vi "Untitled 2.vi"(8 "error in (no error)":errorcluster) -> ()   [LabVIEW 2015]
uses:
  Camera Types.ctl
  <vilib>/Rock Robotics/WPI/Camera/WPI_CameraImageSize.ctl
  <vilib>/Rock Robotics/WPI/Camera/WPI_CameraWhite Balance Values.ctl
  <vilib>/Rock Robotics/WPI/Camera/WPI_CameraExposure Values.ctl
  <vilib>/Rock Robotics/WPI/Camera/WPI_CameraFrameRate.ctl
  Global 2.vi
  Robot Global Data.vi
  Global 1.vi
  <vilib>/vision/NI_Vision_Development_Module.lvlib
panel:
  in  "Cluster":T1={"Hue"={105.0, 150.0}, "Sat"={191.0, 255.0}, "Val"={173.0, 255.0}}
  in  "Image Size":T2=enum."320x240"
  out "Original Image":T3(plugin-control)
  out "Masked":T3(plugin-control)
  out "Qualified Particles":i32
  out "Sorted Particle Scores":T4(array[cluster]) {"Moment Factor" format="%#_3g"; "Aspect Ratio" format="%#_3g"; "Area to CH" format="%#_3g"; "X" format="%#_3g"; "Y" format="%#_3g"}
  in  "Annotate":bool=TRUE
  in  "Annotation Limit":dbl=75.0
  out "Detected Targets":T5(array[cluster]) {"Normalized Rect"."Numeric 5" format="%#_2g"; "Normalized Rect"."Numeric 3" format="%#_2g"; "Normalized Rect"."Numeric 2" format="%#_2g"; "Normalized Rect"."Numeric" format="%#_2g"}
  in  "Aspect Ratio Fudge Factor":dbl=1.0
  out "Highest Avg Score":dbl format="%#_3g"
  in  "Min Score Threshold":i32=70
  in  "Camera Type":T6=enum."MS HD3000 square"
  in  "Emphasize Limit Tests":bool=TRUE
  in  "Std Devs for Calibration":cluster{"H":dbl, "S":dbl, "V":dbl}={"H"=4.0, "S"=6.0, "V"=6.0}
  # "Density Profile"
  # "x"
  # "y"
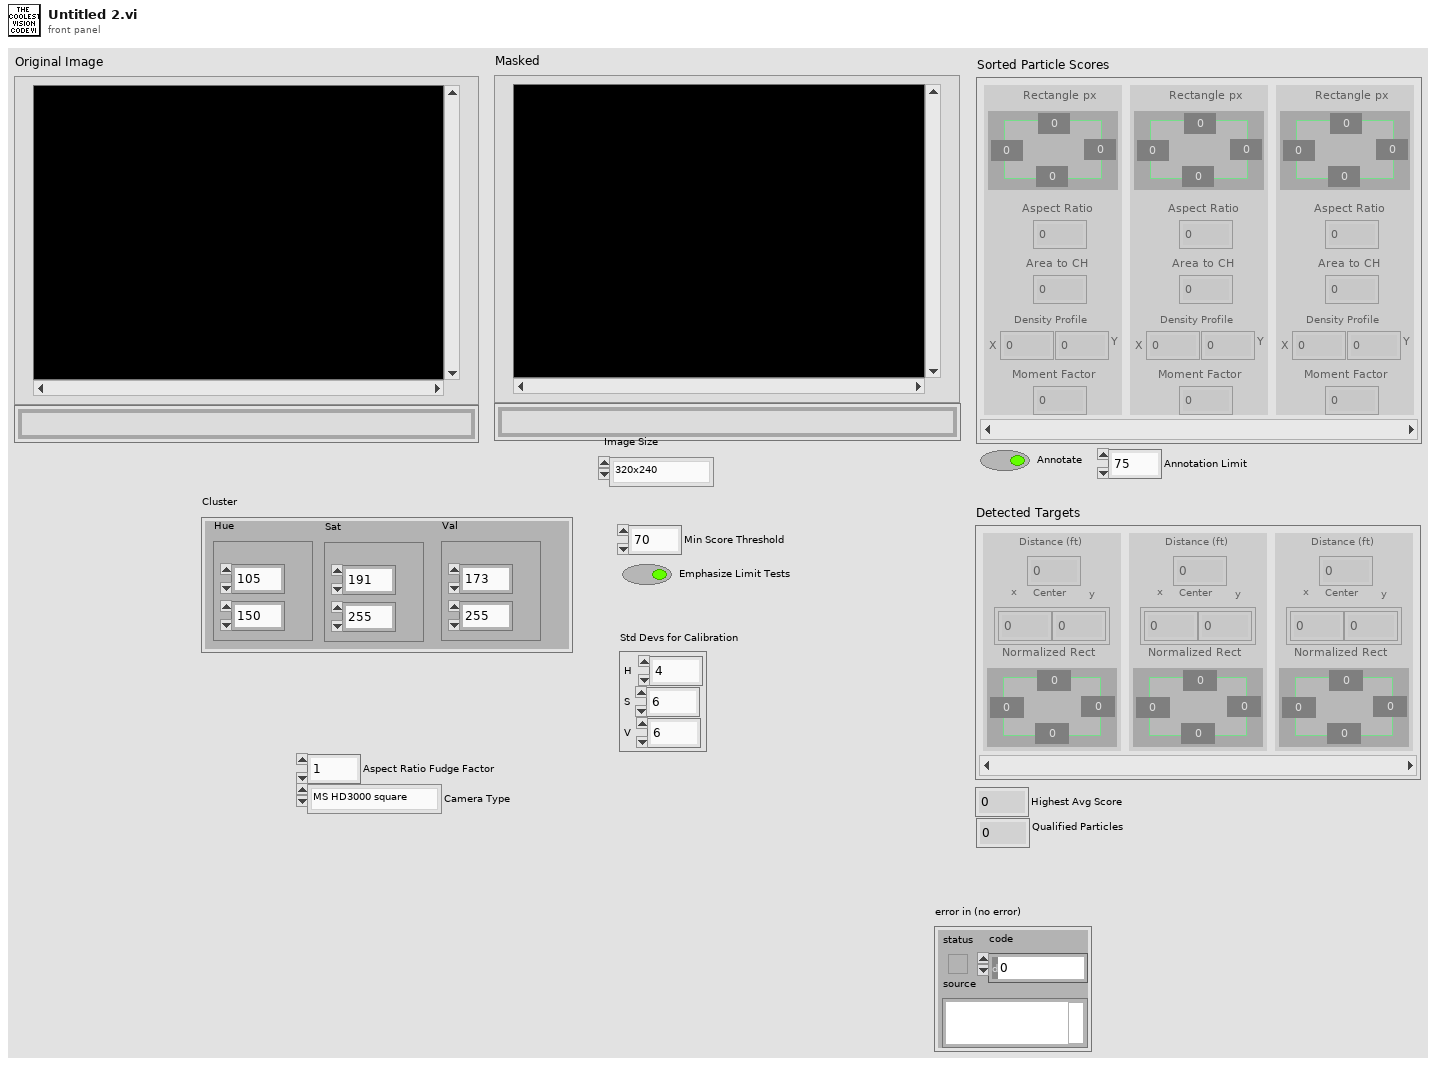
[diagram p1: front panel]
types:
  T1 = cluster{"Hue":cluster{dbl, dbl}, "Sat":cluster{dbl, dbl}, "Val":cluster{dbl, dbl}}
  T2 = typedef "WPI_CameraImageSize.ctl" = enum16{"640x480", "320x240", "160x120", "Custom"}
  T3 = typedef "IMAQ Image.ctl" = refnum<image>
  T4 = cluster{"Rectangle px":cluster{"Numeric":dbl, "Numeric 2":dbl, "Numeric 3":dbl, "Numeric 5":dbl}, "Aspect Ratio":dbl, "Area to CH":dbl, "X":dbl, "Y":dbl, "Moment Factor":dbl}[]
  T5 = cluster{"Distance (ft)":dbl, "Center":cluster{dbl, dbl}, "Normalized Rect":cluster{"Numeric":dbl, "Numeric 2":dbl, "Numeric 3":dbl, "Numeric 5":dbl}}[]
  T6 = typedef "Camera Types.ctl" = enum16{"206", "1011", "1013", "MS HD3000 square", "MS HD3000 640x480"}
  T7 = typedef "WPI_CameraFrameRate.ctl" = u32
  T8 = typedef "WPI_CameraExposure Values.ctl" = enum16{"Auto", "Flicker-free 50 Hz", "Flicker-free 60 Hz", "Hold current", "Custom"}
  T9 = typedef "WPI_CameraWhite Balance Values.ctl" = enum16{"Auto", "Fixed indoor", "Fixed outdoor 1", "Fixed outdoor 2", "Fixed fluorescent 1", "Fixed fluorescent 2", "Hold current", "Custom"}
  T10 = typedef "Particle Parameters" = i32
  T11 = typedef "Image Type" = u32
  T12 = typedef "WPI_CameraDevRef.ctl" = cluster{"Camera Address":string, "CameraStatus":errorcluster}
  T13 = cluster{cluster{dbl, dbl}, cluster{dbl, dbl}, cluster{dbl, dbl}}
  T14 = cluster{"Bounding box":cluster{"left":dbl, "top":dbl, "right":dbl, "bottom":dbl}, "Aspect Ratio":dbl, "Area to CH":dbl, "X Mask":dbl, "Y Mask":dbl, "Moment":dbl}[]
  T15 = cluster{"Rectangle":cluster{"Numeric":dbl, "Numeric 2":dbl, "Numeric 3":dbl, "Numeric 5":dbl}, "L":dbl, "Area to CH":dbl, "X":dbl, "Y":dbl, "Moment Factor":dbl}[]
  T16 = cluster{"Found Targets[0]":cluster{"Distance (ft)":dbl, "Center":cluster{dbl, dbl}, "Normalized Rect":cluster{"Numeric":dbl, "Numeric 2":dbl, "Numeric 3":dbl, "Numeric 5":dbl}}, "Found Targets[1]":cluster{"Distance (ft)":dbl, "Center":cluster{dbl, dbl}, "Normalized Rect":cluster{"Numeric":dbl, "Numeric 2":dbl, "Numeric 3":dbl, "Numeric 5":dbl}}, "Found Targets[2]":cluster{"Distance (ft)":dbl, "Center":cluster{dbl, dbl}, "Normalized Rect":cluster{"Numeric":dbl, "Numeric 2":dbl, "Numeric 3":dbl, "Numeric 5":dbl}}, "Found Targets[3]":cluster{"Distance (ft)":dbl, "Center":cluster{dbl, dbl}, "Normalized Rect":cluster{"Numeric":dbl, "Numeric 2":dbl, "Numeric 3":dbl, "Numeric 5":dbl}}, "Found Targets[4]":cluster{"Distance (ft)":dbl, "Center":cluster{dbl, dbl}, "Normalized Rect":cluster{"Numeric":dbl, "Numeric 2":dbl, "Numeric 3":dbl, "Numeric 5":dbl}}, "Found Targets[5]":cluster{"Distance (ft)":dbl, "Center":cluster{dbl, dbl}, "Normalized Rect":cluster{"Numeric":dbl, "Numeric 2":dbl, "Numeric 3":dbl, "Numeric 5":dbl}}, "Found Targets[6]":cluster{"Distance (ft)":dbl, "Center":cluster{dbl, dbl}, "Normalized Rect":cluster{"Numeric":dbl, "Numeric 2":dbl, "Numeric 3":dbl, "Numeric 5":dbl}}, "Found Targets[7]":cluster{"Distance (ft)":dbl, "Center":cluster{dbl, dbl}, "Normalized Rect":cluster{"Numeric":dbl, "Numeric 2":dbl, "Numeric 3":dbl, "Numeric 5":dbl}}, "Found Targets[8]":cluster{"Distance (ft)":dbl, "Center":cluster{dbl, dbl}, "Normalized Rect":cluster{"Numeric":dbl, "Numeric 2":dbl, "Numeric 3":dbl, "Numeric 5":dbl}}}
  T17 = cluster{"Distance (ft)":dbl, "Center":cluster{dbl, dbl}, "Normalized Rect":cluster{"Numeric":dbl, "Numeric 2":dbl, "Numeric 3":dbl, "Numeric 5":dbl}}
  T18 = cluster{"Numeric":dbl, "Numeric 2":dbl, "Numeric 3":dbl, "Numeric 5":dbl}
  T19 = cluster{"Distance (ft)":dbl, cluster{dbl, dbl}, "Normalized Rect":cluster{"Numeric":dbl, "Numeric 2":dbl, "Numeric 3":dbl, "Numeric 5":dbl}}
  T20 = cluster{cluster{"Distance (ft)":dbl, cluster{dbl, dbl}, "Normalized Rect":cluster{"Numeric":dbl, "Numeric 2":dbl, "Numeric 3":dbl, "Numeric 5":dbl}}, cluster{"Distance (ft)":dbl, cluster{dbl, dbl}, "Normalized Rect":cluster{"Numeric":dbl, "Numeric 2":dbl, "Numeric 3":dbl, "Numeric 5":dbl}}, cluster{"Distance (ft)":dbl, cluster{dbl, dbl}, "Normalized Rect":cluster{"Numeric":dbl, "Numeric 2":dbl, "Numeric 3":dbl, "Numeric 5":dbl}}, "Found Targets[3]":cluster{"Distance (ft)":dbl, "Center":cluster{dbl, dbl}, "Normalized Rect":cluster{"Numeric":dbl, "Numeric 2":dbl, "Numeric 3":dbl, "Numeric 5":dbl}}, "Found Targets[4]":cluster{"Distance (ft)":dbl, "Center":cluster{dbl, dbl}, "Normalized Rect":cluster{"Numeric":dbl, "Numeric 2":dbl, "Numeric 3":dbl, "Numeric 5":dbl}}, "Found Targets[5]":cluster{"Distance (ft)":dbl, "Center":cluster{dbl, dbl}, "Normalized Rect":cluster{"Numeric":dbl, "Numeric 2":dbl, "Numeric 3":dbl, "Numeric 5":dbl}}, "Found Targets[6]":cluster{"Distance (ft)":dbl, "Center":cluster{dbl, dbl}, "Normalized Rect":cluster{"Numeric":dbl, "Numeric 2":dbl, "Numeric 3":dbl, "Numeric 5":dbl}}, "Found Targets[7]":cluster{"Distance (ft)":dbl, "Center":cluster{dbl, dbl}, "Normalized Rect":cluster{"Numeric":dbl, "Numeric 2":dbl, "Numeric 3":dbl, "Numeric 5":dbl}}, "Found Targets[8]":cluster{"Distance (ft)":dbl, "Center":cluster{dbl, dbl}, "Normalized Rect":cluster{"Numeric":dbl, "Numeric 2":dbl, "Numeric 3":dbl, "Numeric 5":dbl}}}
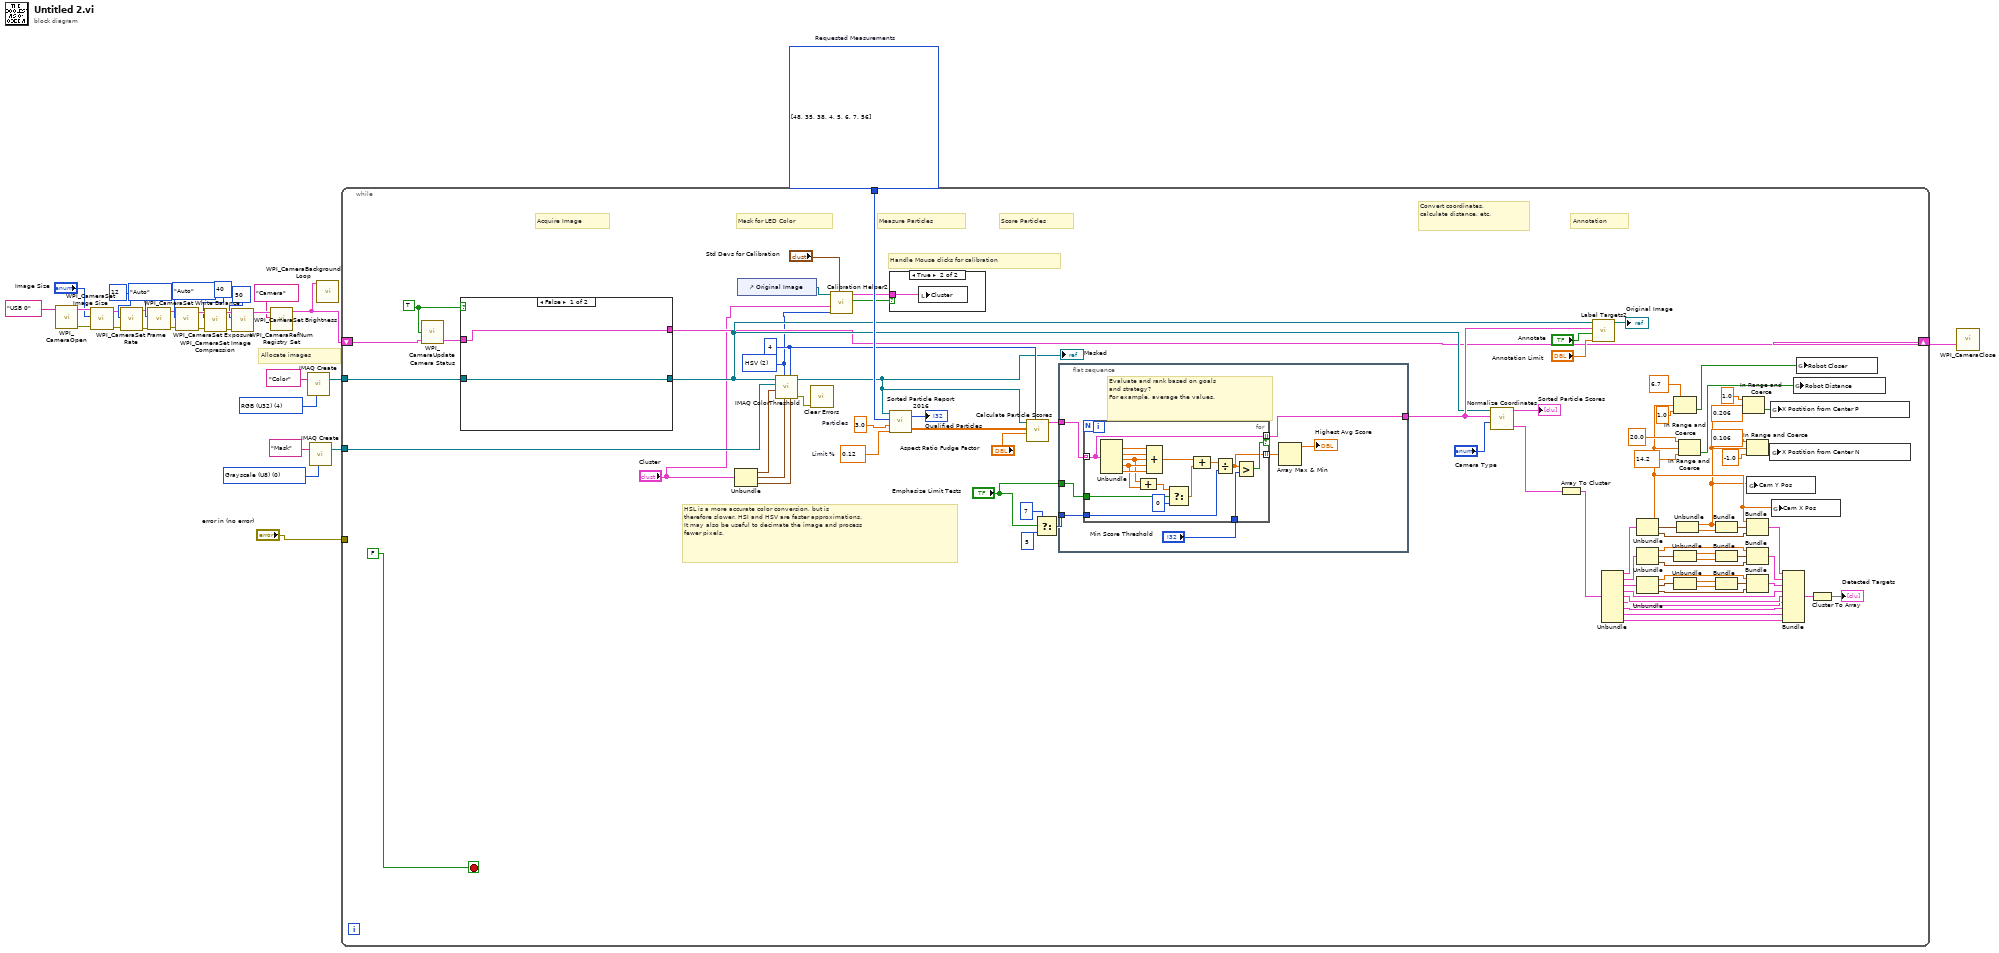
[diagram p0: block diagram]
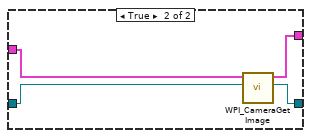
[diagram p3: hidden frame]
diagram:
  w25 = T10[] [48, 35, 38, 4, 5, 6, 7, 56] items=["Center of Mass X", "Center of Mass Y", "First Pixel X", "First Pixel Y", "Bounding Rect Left", "Bounding Rect Top", "Bounding Rect Right", "Bounding Rect Bottom", "Max Feret Diameter Start X", "Max Feret Diameter Start Y", "Max Feret Diameter End X", "Max Feret Diameter End Y", "Max Horiz. Segment Length Left", "Max Horiz. Segment Length Right", "Max Horiz. Segment Length Row", "-", "Bounding Rect Width", "Bounding Rect Height", "Bounding Rect Diagonal", "Perimeter", "Convex Hull Perimeter", "Holes' Perimeter", "Max Feret Diameter", "Equivalent Ellipse Major Axis", "Equivalent Ellipse Minor Axis", "Equivalent Ellipse Minor Axis (Feret)", "Equivalent Rect Long Side", "Equivalent Rect Short Side", "Equivalent Rect Diagonal", "Equivalent Rect Short Side (Feret)", "Average Horiz. Segment Length", "Average Vert. Segment Length", "Hydraulic Radius", "Waddel Disk Diameter", "-", "Area", "Holes' Area", "Particle & Holes' Area", "Convex Hull Area", "Image Area", "-", "Number of Holes", "Number of Horiz. Segments", "Number of Vert. Segments", "-", "Orientation", "Max Feret Diameter Orientation", "-", "% Area/Image Area", "% Area/(Particle & Holes' Area)", "Ratio of Equivalent Ellipse Axes", "Ratio of Equivalent Rect Sides", "-", "Elongation Factor", "Compactness Factor", "Heywood Circularity Factor", "Type Factor", "-", "Sum X", "Sum Y", "Sum XX", "Sum XY", "Sum YY", "Sum XXX", "Sum XXY", "Sum XYY", "Sum YYY", "-", "Moment of Inertia XX", "Moment of Inertia XY", "Moment of Inertia YY", "Moment of Inertia XXX", "Moment of Inertia XXY", "Moment of Inertia XYY", "Moment of Inertia YYY", "Norm. Moment of Inertia XX", "Norm. Moment of Inertia XY", "Norm. Moment of Inertia YY", "Norm. Moment of Inertia XXX", "Norm. Moment of Inertia XXY", "Norm. Moment of Inertia XYY", "Norm. Moment of Inertia YYY", "Hu Moment 1", "Hu Moment 2", "Hu Moment 3", "Hu Moment 4", "Hu Moment 5", "Hu Moment 6", "Hu Moment 7"]  # Requested Measurements
  w28 = T11 0 items=["Grayscale (U8)", "Grayscale (I16)", "Grayscale (SGL)", "Complex (CSG)", "RGB (U32)", "HSL (U32)", "RGB (U64)", "Grayscale (U16)"] ("Image Type")
  w30 = T11 4 items=["Grayscale (U8)", "Grayscale (I16)", "Grayscale (SGL)", "Complex (CSG)", "RGB (U32)", "HSL (U32)", "RGB (U64)", "Grayscale (U16)"] ("Image Type")
  # "Allocate images"
  n1 = call <vilib>:"WPI_CameraOpen.vi"("Camera Address"="USB 0") -> ("error out"=w11:errorcluster, "CameraDevRef"=w24:T12)  [unwired: 9 in]
  n2 = call <vilib>:"WPI_CameraSet Image Size.vi"("error in (no error)"=w11, "Image Size"="Image Size", "CameraDevRef"=w24) -> ("error out"=w10:errorcluster, "CameraDevRef Out"=w19:T12)  [unwired: 1 in, 6 out]
  n3 = call <vilib>:"WPI_CameraSet Frame Rate.vi"("error in (no error)"=w10, "Frame Rate (fps)"=T7 12, "CameraDevRef"=w19) -> ("error out"=w9:errorcluster, "CameraDevRef Out"=w17:T12)  [unwired: 7 out]
  n4 = call <vilib>:"WPI_CameraSet White Balance.vi"("error in (no error)"=w9, "White Balance"=WPI_CameraWhite_Balance_Values."Auto", "CameraDevRef"=w17) -> ("error out"=w8:errorcluster, "CameraDevRef Out"=w18:T12)  [unwired: 1 in, 6 out]
  n5 = call <vilib>:"WPI_CameraSet Exposure.vi"("error in (no error)"=w8, "Exposure"=WPI_CameraExposure_Values."Auto", "CameraDevRef"=w18) -> ("error out"=w7:errorcluster, "CameraDevRef Out"=w15:T12)  [unwired: 1 in, 6 out]
  n6 = call <vilib>:"WPI_CameraSet Image Compression.vi"("error in (no error)"=w7, "Compression"=40, "CameraDevRef"=w15) -> ("error out"=w6:errorcluster, "CameraDevRef Out"=w16:T12)  [unwired: 7 out]
  n7 = call <vilib>:"WPI_CameraSet Brightness.vi"("error in (no error)"=w6, "Brightness"=50, "CameraDevRef"=w16) -> ("CameraDevRef Out"=w4:T12)  [unwired: 8 out]
  n8 = call <vilib>:"WPI_CameraRefNum Registry Set.vi"("refnum name"="Camera", "CameraDevRef"=w4) -> ("CameraDevRef"=w1:T12)  [unwired: 8 in, 1 out]
  n9 = call "IMAQ Create"("Image Name"="Color", "Image Type"=w30) -> ("New Image"=w29:T3)  [unwired: 2 in, 2 out]
  n10 = call "IMAQ Create"("Image Name"="Mask", "Image Type"=w28) -> ("New Image"=w26:T3)  [unwired: 2 in, 2 out]
  n11 = call <vilib>:"WPI_CameraBackground Loop.vi"("CameraDevRef"=w1) -> ()  [unwired: 11 in]
  n12 = while {
    tunnel: w29 -> [w114]
    tunnel: w26 -> [w112]
    tunnel: w25 -> [w108]
    tunnel: "error in (no error)" -> [_]
    shift-right: [w85] -> w2
    shift-left: w1 -> [w84]
    stop <- FALSE stop-if-true
    w86 = TRUE
    w101 = 4 ("Replace Value")
    w104 = 0.12  # Limit %
    w107 = 3.0  # Particles
    w79 = u16 2 items=["RGB", "HSL", "HSV", "HSI"] ("Color Mode")
    # "Handle Mouse clicks for calibration"
    # "Measure Particles"
    # "Convert coordinates,\ncalculate distance, etc."
    # "Annotation"
    # "Score Particles"
    # "Mask for LED Color"
    # "Acquire Image"
    # "HSL is a more accurate color conversion, but is\ntherefore slower. HSI and HSV are faster approximations.\nIt may also be useful to decimate the image and process\nfewer pixels."
    n13 = call <vilib>:"WPI_CameraUpdate Camera Status.vi"("CameraDevRef In"=w84, "Enable Vision"=w86) -> ("CameraDevRef Out"=w87:T12)  [unwired: 3 in]
    n14 = case shown="False" w86 {
      tunnel: [w139 w143] -> w89
      tunnel: w114 -> [w139 w144]
      tunnel: w87 -> [w140 w142]
      tunnel: [w140 w141] -> w85
      frame False {
      }
      frame True {
        n15 = call <vilib>:"WPI_CameraGet Image.vi"("Image"=w144, "CameraDevRef"=w142) -> ("Image Out"=w143:T3, "CameraDevRef Out"=w141:T12)  [unwired: 7 in, 1 out]
      }
    }
    n16 = Unbundle("Cluster") -> ("Hue"=w111:cluster{dbl, dbl}, "Sat"=w110:cluster{dbl, dbl}, "Val"=w109:cluster{dbl, dbl})
    n17 = control-ref of="Original Image"() -> (w80:refnum<vi>)
    n18 = call "IMAQ ColorThreshold"("Blue or Luma or Val or Inten Range"=w109, "Replace Value"=w101, "Green or Sat Range"=w110, "Color Mode"=w79, "Red or Hue Range"=w111, "Image Dst"=w112, "Image Src"=w89) -> ("error out"=w93:errorcluster, "Image Dst Out"=w94:T3)  [unwired: 3 in]
    "Masked" <- w94
    n19 = call <vilib>:"Clear Errors.vi"("error in (no error)"=w93) -> ()  [unwired: 5 in, 2 out]
    n20 = call "Calibration Helper2.vi"("Std Devs"="Std Devs for Calibration", "Color Mode"=w79, "Color Components"="Cluster", "Image Ctl Refnum"=w80) -> ("Changed"=w83:bool, "output color"=w81:T13)  [unwired: 6 in]
    n21 = case shown="True" w83 {
      tunnel: w81 -> [_ w115]
      frame False {
      }
      frame True {
        n22 = local write "Cluster"(w115) -> ()
      }
    }
    n23 = call "Sorted Particle Report 2016.vi"("Min Area Size %"=w104, "Particle Count Limit"=w107, "Pixel Measurements"=w108, "Image in"=w94) -> ("Sorted Data"=w105:dbl[][], "Particles"=→"Qualified Particles":i32)
    n24 = call "Calculate Particle Scores.vi"("Pixel Value"=w101, "Aspect Fudge Factor"="Aspect Ratio Fudge Factor", "Sorted Data"=w105, "Image in"=w94) -> ("Scores"=w97:T14)  [unwired: 7 in]
    n25 = Select(t=7, s="Emphasize Limit Tests", f=5) -> (s? t:f=w90:i32)
    n26 = flat-sequence {
      tunnel: w97 -> [w121]
      tunnel: [w122] -> w95
      tunnel: w90 -> [w118]
      tunnel: "Emphasize Limit Tests" -> [w116]
      frame #0 {
        # "Evaluate and rank based on goals\nand strategy?\nFor example, average the values."
        n27 = for {
          tunnel: w121 -> [w136] mode=indexing
          tunnel: [w136] -> w122 mode=indexing if=w135
          tunnel: [w134] -> w120 mode=indexing
          tunnel: w118 -> [w133]
          tunnel: "Min Score Threshold" -> [w132]
          tunnel: w116 -> [w125]
          n28 = Unbundle(w136) -> ("Aspect Ratio"=w138:dbl, "Area to CH"=w137:dbl, "X Mask"=w127:dbl, "Y Mask"=w128:dbl, "Moment"=w129:dbl)  [unwired: 1 out]
          n29 = Compound Arithmetic op=ADD(w127, w128) -> (w126:dbl)
          n30 = Compound Arithmetic op=ADD(w138, w137, w127, w128, w129) -> (w131:dbl)
          n31 = Select(t=w126, s=w125, f=0) -> (s? t:f=w124:dbl)
          n32 = Compound Arithmetic op=ADD(w131, w124) -> (w130:dbl)
          n33 = Divide(x=w130, y=w133) -> (x/y=w134:dbl)
          n34 = Greater?(x=w134, y=w132) -> (0:w135:bool)
        }
        n35 = Array Max & Min(array=w120) -> (max value=→"Highest Avg Score":dbl)  [unwired: 3 out]
      }
    }
    n36 = call "Normalize Coordinates.vi"("Camera Type"="Camera Type", "Targets"=w95, "Image in"=w89) -> ("Found Targets"=w77:T5, "Sorted Scores"=→"Sorted Particle Scores":T15)  [unwired: 7 in]
    n37 = Array To Cluster(array=w77) -> (cluster=w76:T16)
    n38 = call "Label Targets2.vi"("Score Threshold"="Annotation Limit", "Annotate"="Annotate", "Targets"=w95, "Image in"=w89) -> ("Image out"=→"Original Image":T3)  [unwired: 7 in]
    n39 = Unbundle(w76) -> ("Found Targets[0]"=w75:T17, "Found Targets[1]"=w72:T17, "Found Targets[2]"=w73:T17, "Found Targets[3]"=w45:T17, "Found Targets[4]"=w44:T17, "Found Targets[5]"=w43:T17, "Found Targets[6]"=w42:T17, "Found Targets[7]"=w41:T17, "Found Targets[8]"=w40:T17)
    n40 = Unbundle(w75) -> ("Distance (ft)"=w33:dbl, "Center"=w74:cluster{dbl, dbl}, "Normalized Rect"=w59:T18)
    n41 = Unbundle(w72) -> ("Distance (ft)"=w58:dbl, "Center"=w71:cluster{dbl, dbl}, "Normalized Rect"=w60:T18)
    n42 = Unbundle(w73) -> ("Distance (ft)"=w57:dbl, "Center"=w70:cluster{dbl, dbl}, "Normalized Rect"=w61:T18)
    n43 = In Range and Coerce(upper limit=6.7, x=w33, lower limit=1.0) -> (In Range?=w50:bool)  [unwired: 1 out]
    n44 = Unbundle(w71) -> (w69:dbl, w68:dbl)
    n45 = Unbundle(w70) -> (w67:dbl, w66:dbl)
    n46 = Unbundle(w74) -> (w32:dbl, w51:dbl)
    n47 = In Range and Coerce(upper limit=20.0, x=w33, lower limit=14.2) -> (In Range?=w52:bool)  [unwired: 1 out]
    n48 = Bundle(w32, w51) -> (w64:cluster{dbl, dbl})  [unwired: 1 in]
    n49 = Bundle(w69, w68) -> (w63:cluster{dbl, dbl})  [unwired: 1 in]
    n50 = Bundle(w67, w66) -> (w62:cluster{dbl, dbl})  [unwired: 1 in]
    n51 = In Range and Coerce(upper limit=1.0, x=w32, lower limit=0.206) -> (In Range?=w49:bool)  [unwired: 1 out]
    n52 = In Range and Coerce(upper limit=0.106, x=w32, lower limit=-1.0) -> (In Range?=w48:bool)  [unwired: 1 out]
    n53 = Bundle("Distance (ft)"=w33, w64, "Normalized Rect"=w59) -> (w56:T19)  [unwired: 1 in]
    n54 = Bundle("Distance (ft)"=w58, w63, "Normalized Rect"=w60) -> (w55:T19)  [unwired: 1 in]
    n55 = Bundle("Distance (ft)"=w57, w62, "Normalized Rect"=w61) -> (w54:T19)  [unwired: 1 in]
    n56 = global write "Global 2.vi" "Cam Y Pos"(w32) -> ()
    n57 = global write "Robot Global Data.vi" "X Postition from Center N"(w48) -> ()
    n58 = global write "Robot Global Data.vi" "X Postition from Center P"(w49) -> ()
    n59 = global write "Global 1.vi" "Cam X Pos"(w33) -> ()
    n60 = Bundle(w56, w55, w54, "Found Targets[3]"=w45, "Found Targets[4]"=w44, "Found Targets[5]"=w43, "Found Targets[6]"=w42, "Found Targets[7]"=w41, "Found Targets[8]"=w40) -> (w65:T20)  [unwired: 1 in]
    n61 = global write "Robot Global Data.vi" "Robot Distance"(w52) -> ()
    n62 = global write "Robot Global Data.vi" "Robot Closer"(w50) -> ()
    n63 = Cluster To Array(cluster=w65) -> (array=→"Detected Targets":T5)
  }
  n64 = call <vilib>:"WPI_CameraClose.vi"("CameraDevRef"=w2) -> ()  [unwired: 10 in, 1 out]
